vi "Rotator Status String.vi"(10 "VI Name":string="PS Control.vi") -> (0 "error out":errorcluster, 1 "Status String":string)   [LabVIEW 2025]
doc: "Author: Scott Hannahs <sth@magnet.fsu.edu>\n\nThis software is licensed for use under the “MIT License\"\nCopyright (c) 2025 Scott Hannahs, sth@sth@magnet.sthnet.net\n\nPermission is hereby granted, free of charge, to any person obtaining a copy of this software and associated documentation files (the \"Software\"), to deal in the Software without restriction, including without limitation the rights to use, copy, modify, merge, publish, distribute, sublicense, and/or sell copies of the Software, and to permit persons to whom the Software is furnished to do so, subject to the following conditions: The above copyright notice and this permission notice shall be included in all copies or substantial portions of the Software.\n\nTHE SOFTWARE IS PROVIDED \"AS IS\", WITHOUT WARRANTY OF ANY KIND, EXPRESS OR IMPLIED, INCLUDING BUT NOT LIMITED TO THE WARRANTIES OF MERCHANTABILITY, FITNESS FOR A PARTICULAR PURPOSE AND NONINFRINGEMENT. IN NO EVENT SHALL THE AUTHORS OR COPYRIGHT HOLDERS BE LIABLE FOR ANY CLAIM, DAMAGES OR OTHER LIABILITY, WHETHER IN AN ACTION OF CONTRACT, TORT OR OTHERWISE, ARISING FROM, OUT OF OR IN CONNECTION WITH THE SOFTWARE OR THE USE OR OTHER DEALINGS IN THE SOFTWARE."
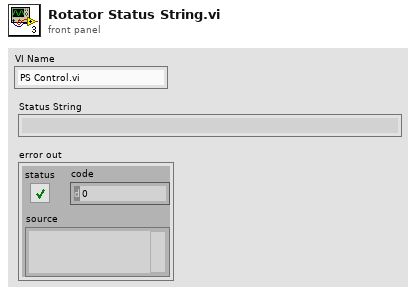
[diagram p1: front panel]
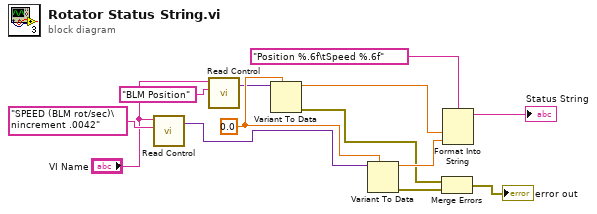
[diagram p0: block diagram]
diagram:
  w6 = 0.0
  n1 = call "Read Control.vi"("VI Name"="VI Name", "Control Name"="SPEED (BLM rot/sec)\nincrement .0042") -> ("Value"=w4:variant)  [unwired: 3 in, 1 out]
  n2 = call "Read Control.vi"("VI Name"="VI Name", "Control Name"="BLM Position") -> ("Value"=w5:variant)  [unwired: 3 in, 1 out]
  n3 = Variant To Data(type=w6, Variant=w5) -> (data=w10:dbl, error out=w7:errorcluster)  [unwired: 1 in]
  n4 = Variant To Data(type=w6, Variant=w4) -> (data=w11:dbl, error out=w8:errorcluster)  [unwired: 1 in]
  n5 = Merge Errors(w7, w8) -> (→"error out":errorcluster)
  n6 = Format Into String(format string="Position %.6f\tSpeed %.6f", w10, w11) -> (resulting string=→"Status String":string)  [unwired: 2 in, 1 out]
